vi "createSineSamples.vi"(6 "phase":dbl, 7 "samples":i32, 8 "error in (no error)":errorcluster, 9 "amplitude":dbl, 10 "freq":dbl, 11 "SoundDeviceData in":refnum<class "SoundDeviceData.lvclass">) -> (0 "error out":errorcluster, 1 "phase out":dbl, 2 "sine wave":dbl[](array[numeric]), 3 "SoundDeviceData out":refnum<class "SoundDeviceData.lvclass">)   [LabVIEW 2009, in "DataMappers.lvlib" / "SoundDeviceData.lvclass"]
uses:
  SoundDeviceData.lvclass
  SoundDeviceData.lvclass/SoundDeviceData.ctl
  <vilib>/Analysis/NI_AALBase.lvlib
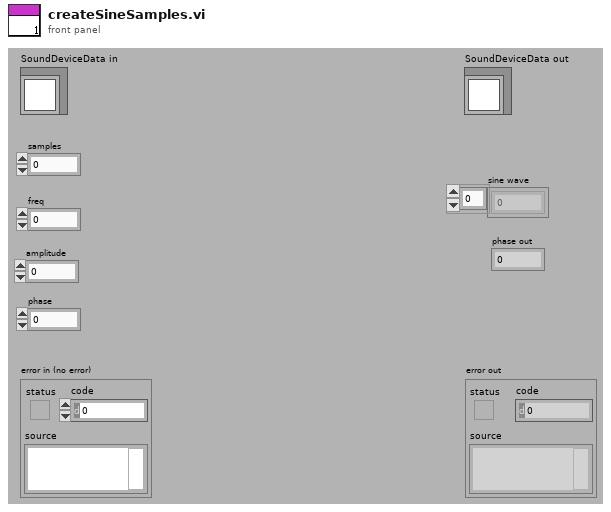
[diagram p1: front panel]
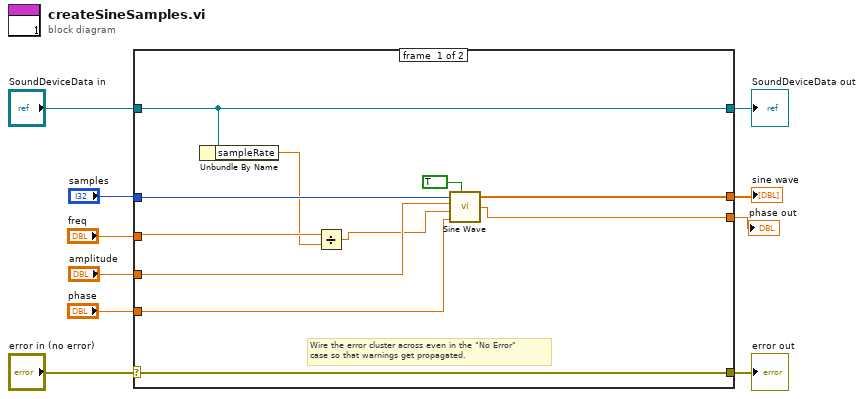
[diagram p0: block diagram]
diagram:
  n1 = case shown="No Error" "error in (no error)" {
    selector: "error in (no error)" -> [w21 w23]
    tunnel: [w21 w23] -> w9
    tunnel: [w19 w22] -> w7
    tunnel: "SoundDeviceData in" -> [w19 w22]
    tunnel: "samples" -> [w20 _]
    tunnel: "freq" -> [w18 _]
    tunnel: "amplitude" -> [w15 _]
    tunnel: "phase" -> [w16 _]
    tunnel: [w12 _] -> w1
    tunnel: [w14 _] -> w2
    frame #0 {
      # "Wire the error cluster across even in the \"No Error\"\ncase so that warnings get propagated."
      n2 = Unbundle By Name(w19) -> ("sampleRate"=w17:dbl)
      n3 = Divide(x=w18, y=w17) -> (x/y=w11:dbl)
      n4 = call <vilib>:"Sine Wave.vi"("samples"=w20, "amplitude"=w15, "frequency"=w11, "phase in"=w16, "reset phase"=TRUE) -> ("sine wave"=w12:dbl[], "phase out"=w14:dbl)  [unwired: 1 out]
    }
    frame #1 {
    }
  }
  "error out" <- w9
  "SoundDeviceData out" <- w7
  "phase out" <- w2
  "sine wave" <- w1
